vi "score generator.vi"(10 "min":dbl=20.0, 11 "max":dbl=80.0) -> (3 "x+y":dbl)   [LabVIEW 2014]
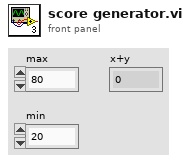
[diagram p1: front panel]
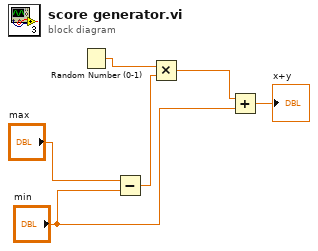
[diagram p0: block diagram]
diagram:
  n1 = Random Number (0-1)() -> (number: 0 to 1=w6:dbl)
  n2 = Subtract(x="max", y="min") -> (x-y=w4:dbl)
  n3 = Multiply(x=w6, y=w4) -> (x*y=w3:dbl)
  n4 = Add(x=w3, y="min") -> (x+y=→"x+y":dbl)
